vi "Untitled 10.vi"() -> ()   [LabVIEW 2017, in "Status Monitor Library.lvlib"]
uses:
  Status Monitor Library.lvlib
  Standalone Status Monitor.vi
panel:
  in  "INI Array":path[](array[path])
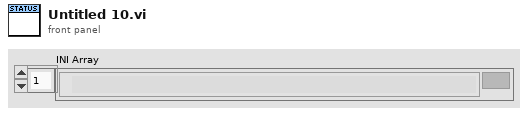
[diagram p1: front panel]
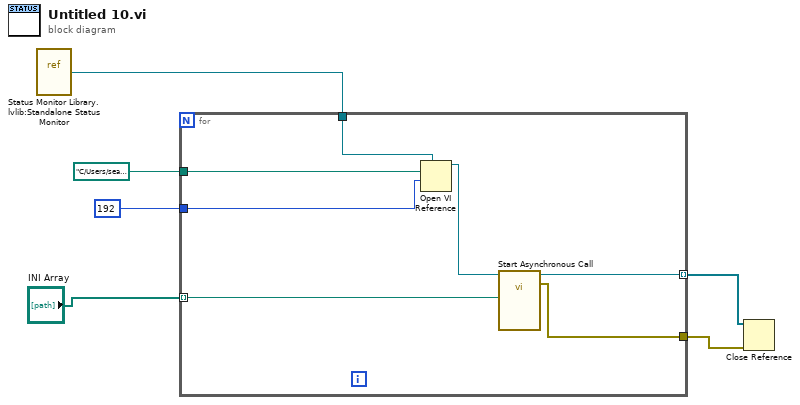
[diagram p0: block diagram]
diagram:
  n1 = vi-ref "Status Monitor Library.lvlib:Standalone Status Monitor.vi"() -> (w5:refnum<vi>)
  n2 = for {
    tunnel: "INI Array" -> [w13] mode=indexing
    tunnel: w5 -> [w12]
    tunnel: path "C:/Users/sean/Documents/Workspace/LabVIEW/Testing/acq400_lv/Source Code/Status Monitor/Standalone Status Monitor.vi" ("vi path") -> [w11]
    tunnel: 192 ("options") -> [w10]
    tunnel: [w8] -> w2 mode=indexing
    tunnel: [w7] -> w1
    n3 = Open VI Reference(type specifier VI Refnum (for type only)=w12, vi path=w11, options=w10) -> (vi reference=w9:refnum<vi>)  [unwired: 3 in, 1 out]
    n4 = call-by-ref "Start Asynchronous Call"(reference=w9, "configuration file path"=w13) -> (reference out=w8:refnum<vi>, error out=w7:errorcluster)  [unwired: 12 in]
  }
  n5 = Close Reference(reference=w2, error in (no error)=w1) -> ()  [unwired: 1 out]
